vi "GyroSensorAquisition.vi"   [LabVIEW 2017]
uses:
  <vilib>/Rock Robotics/WPI/ThirdParty/Phoenix-LabVIEW/Pigeon IMU/CTRE_PigeonIMU_TareType.ctl
  <vilib>/Rock Robotics/WPI/ThirdParty/Phoenix-LabVIEW/Pigeon IMU/CTRE_PigeonIMU_GetTempStateUpTime.vi
  SensorDataGlobal.vi
  <vilib>/Rock Robotics/WPI/ThirdParty/Phoenix-LabVIEW/Pigeon IMU/CTRE_PigeonIMU_GetRawGyro.vi
  <vilib>/Rock Robotics/WPI/ThirdParty/Phoenix-LabVIEW/Pigeon IMU/CTRE_PigeonIMU_GetFusedHeading.vi
types:
  T1 = typedef "CTRE_PigeonIMU_DeviceRef.ctl" = cluster{"DeviceStatus":errorcluster, "Device Number":u8, "Type":T2, "Device ID":u32, "Handle":u64, "UsageFrame":u32, "Library Path":path}
  T2 = typedef "CTRE_PigeonIMU_ConnectionType.ctl" = u32
  T3 = typedef "CTRE_PigeonIMU_CalibrationMode.ctl" = u16
  T4 = typedef "CTRE_PigeonIMU_PigeonState.ctl" = enum16{"NoComm", "Initializing", "Ready", "UserCalibration"}
  T5 = cluster{"CurrentMode":T3, "LastCalError":i32, "CalBooting?":bool, "PigeonState":T4, "UpTime":u32, "Temp. (C)":dbl, "Temp Compensation Event Count":u32, "No Motion Event Count":u32}
  T6 = cluster{"Heading":dbl, "Valid?":bool, "Fusing?":bool}
  T7 = cluster{"X":dbl, "Y":dbl, "Z":dbl, "Magnitude":dbl}
  T8 = typedef "CTRE_PigeonIMU_TareType.ctl" = u8
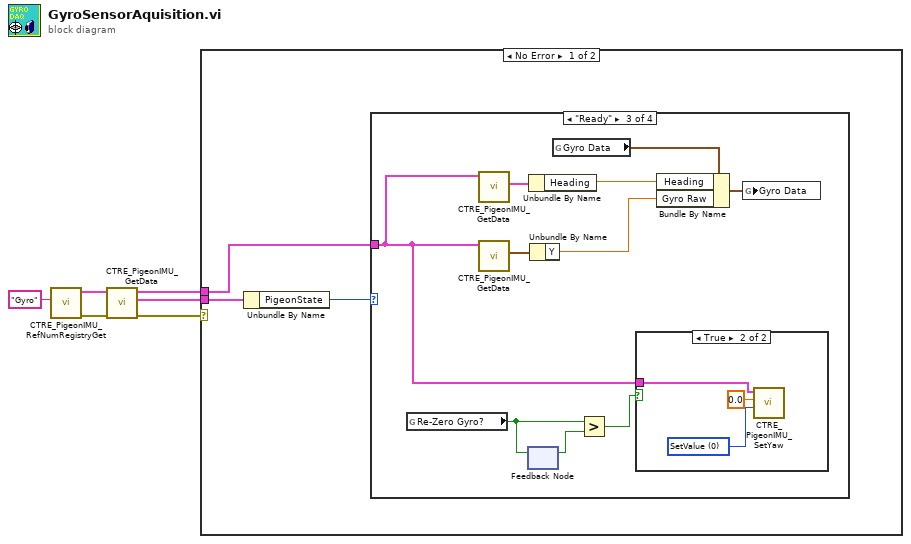
[diagram p0: block diagram]
diagram:
  n1 = call <vilib>:"CTRE_PigeonIMU_RefNumRegistryGet.vi"("refnum name"="Gyro") -> ("error out"=w3:errorcluster, "PigeonIMUDevRef"=w4:T1)  [unwired: 9 in]
  n2 = call-poly <vilib>:"CTRE_PigeonIMU_GetData.vi"("error in (no error)"=w3, "PigeonIMUDevRef"=w4) -> ("error out"=w1:errorcluster, "Temp/State/UpTime"=w6:T5, "PigeonIMUDevRef"=w5:T1)  [unwired: 7 in]
  n3 = case shown="No Error" w1 {
    tunnel: w6 -> [w9 _]
    tunnel: w5 -> [w7 _]
    frame No Error {
      n4 = Unbundle By Name(w9) -> ("PigeonState"=w8:T4)
      n5 = case shown="\"Ready\"" w8 {
        tunnel: w7 -> [_ _ w13 _]
        frame "NoComm", Default {
        }
        frame "Initializing" {
        }
        frame "Ready" {
          n6 = global read "SensorDataGlobal.vi" "Re-Zero Gyro?"() -> (w10:bool)
          n7 = call-poly <vilib>:"CTRE_PigeonIMU_GetData.vi"("PigeonIMUDevRef"=w13) -> ("Fused Heading"=w18:T6)  [unwired: 8 in, 2 out]
          n8 = call-poly <vilib>:"CTRE_PigeonIMU_GetData.vi"("PigeonIMUDevRef"=w13) -> ("Gyro DPS"=w19:T7)  [unwired: 8 in, 2 out]
          n9 = feedback-in #1(w10) -> ()
          n10 = feedback #1() -> (w12:bool)  [unwired: 1 in]
          n11 = Unbundle By Name(w18) -> ("Heading"=w15:dbl)
          n12 = Unbundle By Name(w19) -> ("Y"=w14:dbl)
          n13 = global read "SensorDataGlobal.vi" "Gyro Data"() -> (w16:cluster{"Heading":dbl, "Gyro Raw":dbl})
          n14 = Greater?(x=w10, y=w12) -> (0:w11:bool)
          n15 = case shown="True" w11 {
            tunnel: w13 -> [_ w21]
            frame False {
            }
            frame True {
              w22 = T8 0 items=["SetValue"=0, "AddOffset"=1, "MatchCompass"=2, "SetOffset"=255] ("TareType (SetValue)")
              n16 = call <vilib>:"CTRE_PigeonIMU_SetYaw.vi"("TareType (SetValue)"=w22, "Value"=0.0, "PigeonIMUDevRef"=w21) -> ()  [unwired: 7 in, 2 out]
            }
          }
          n17 = Bundle By Name(cluster=w16, "Heading"=w15, "Gyro Raw"=w14) -> (w17:cluster{"Heading":dbl, "Gyro Raw":dbl})
          n18 = global write "SensorDataGlobal.vi" "Gyro Data"(w17) -> ()
        }
        frame "UserCalibration" {
        }
      }
    }
    frame Error {
    }
  }
